vi "snmpget.vi"(8 "error in (no error)":errorcluster, 9 "OID":string=".1.3.6.1.4.1.3808.1.1.3.3.3.1.1.4.1 ", 10 "community":string="private", 11 "IP / Hostname":string="172.20.125.112") -> (0 "error out":errorcluster, 3 "return":string="1\r\n")   [LabVIEW 2021]
panel:
  out "snmpget arguments":string
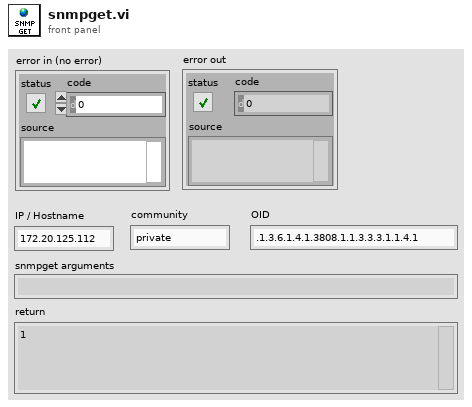
[diagram p1: front panel]
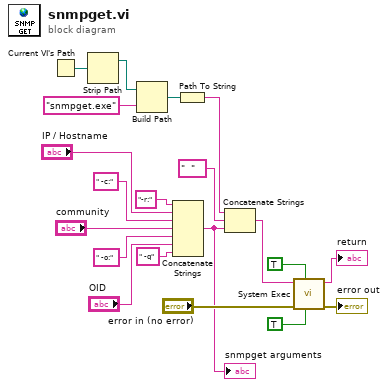
[diagram p0: block diagram]
diagram:
  n1 = Current VI's Path() -> (path=w2:path)
  n2 = Strip Path(path=w2) -> (stripped path=w1:path)  [unwired: 1 out]
  n3 = Build Path(base path=w1, name or relative path="snmpget.exe") -> (appended path=w17:path)
  n4 = Concatenate Strings("-r:" ("string"), "IP / Hostname", " -c:" ("string"), "community", " -o:" ("string"), "OID", " -q" ("string")) -> (w5:string)
  "snmpget arguments" <- w5
  n5 = Path To String(path=w17) -> (string=w19:string)
  n6 = Concatenate Strings(w19, "  " ("standard input"), w5) -> (w14:string)
  n7 = call <vilib>:"System Exec.vi"("run minimized? (F)"=TRUE, "wait until completion? (T)"=TRUE, "error in (no error)"="error in (no error)", "command line"=w14) -> ("error out"=→"error out":errorcluster, "standard output"=→"return":string)  [unwired: 2 in, 4 out]
